vi "1 to 3 Down_movement_v12.vi"(1 "Input pixmap":u8[][](array[numeric]), 2 "start Column":i32) -> (3 "Total point":i32, 4 "moveLog(Row, Col.)":i32[][](array[numeric]), 5 "To:finish Col.":i32, 6 "TapN":dbl)   [LabVIEW 2016]
panel:
  out "RupPoint":dbl[](array[numeric]) format="%_3f"
  out "PointLog":u8[](array[numeric])
  out "min. root p.":u8
  out "3×3 point array":u8[][][](array[numeric])
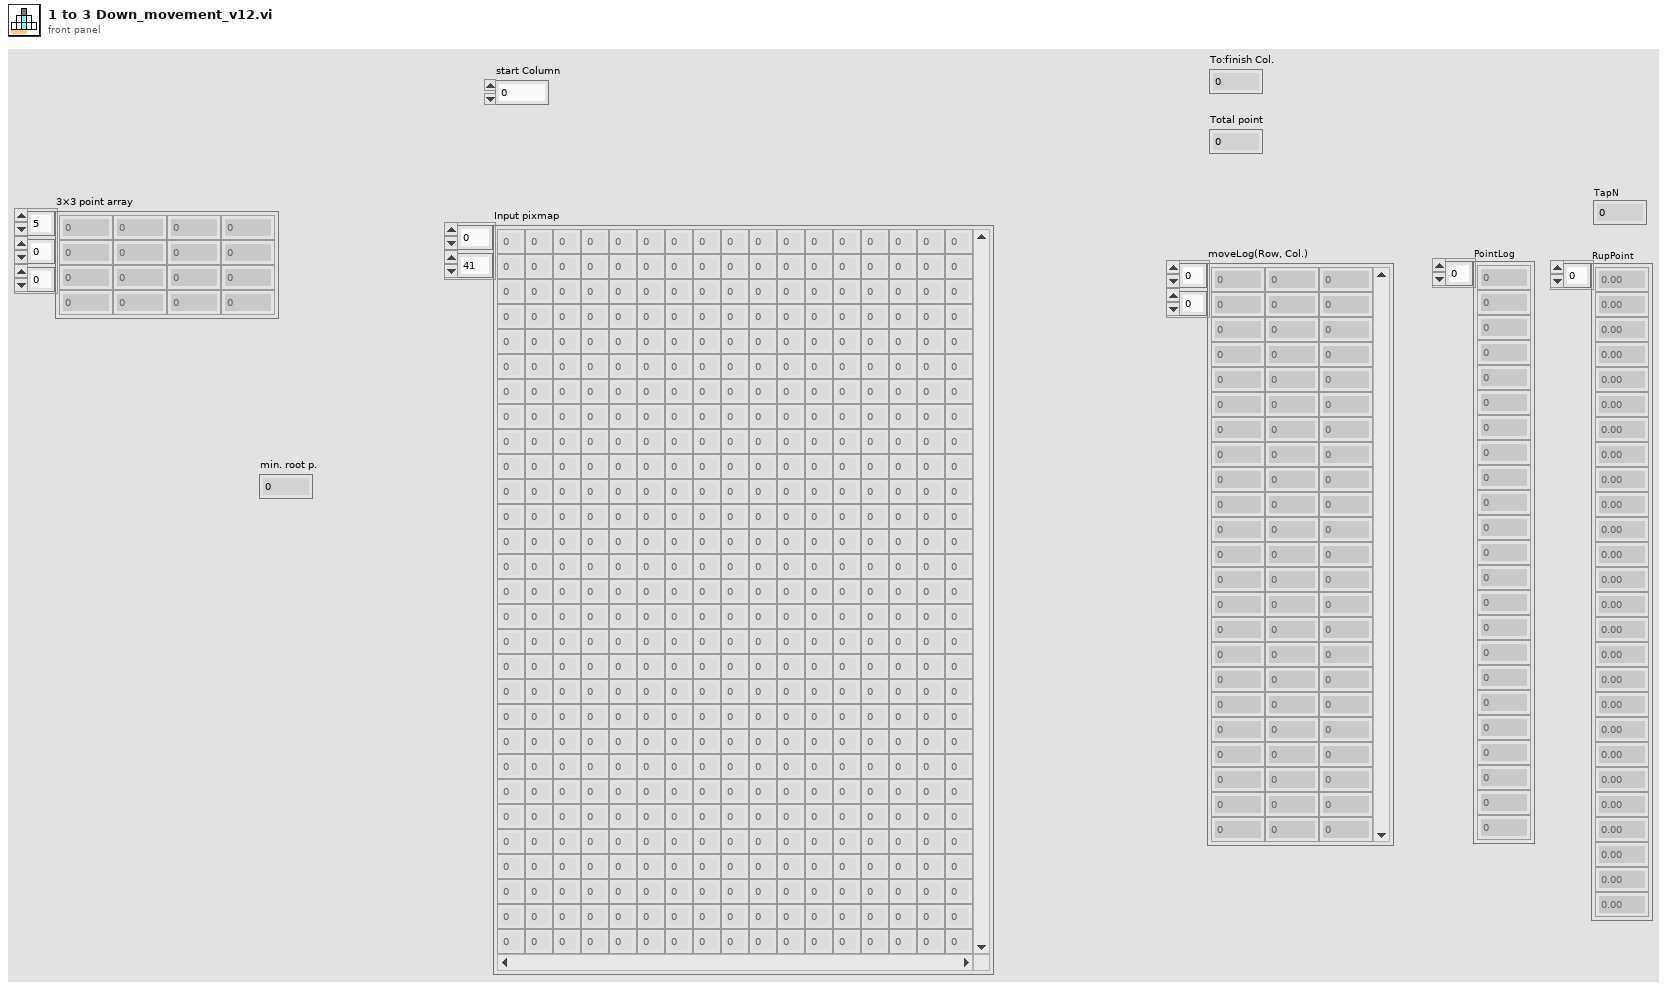
[diagram p1: front panel]
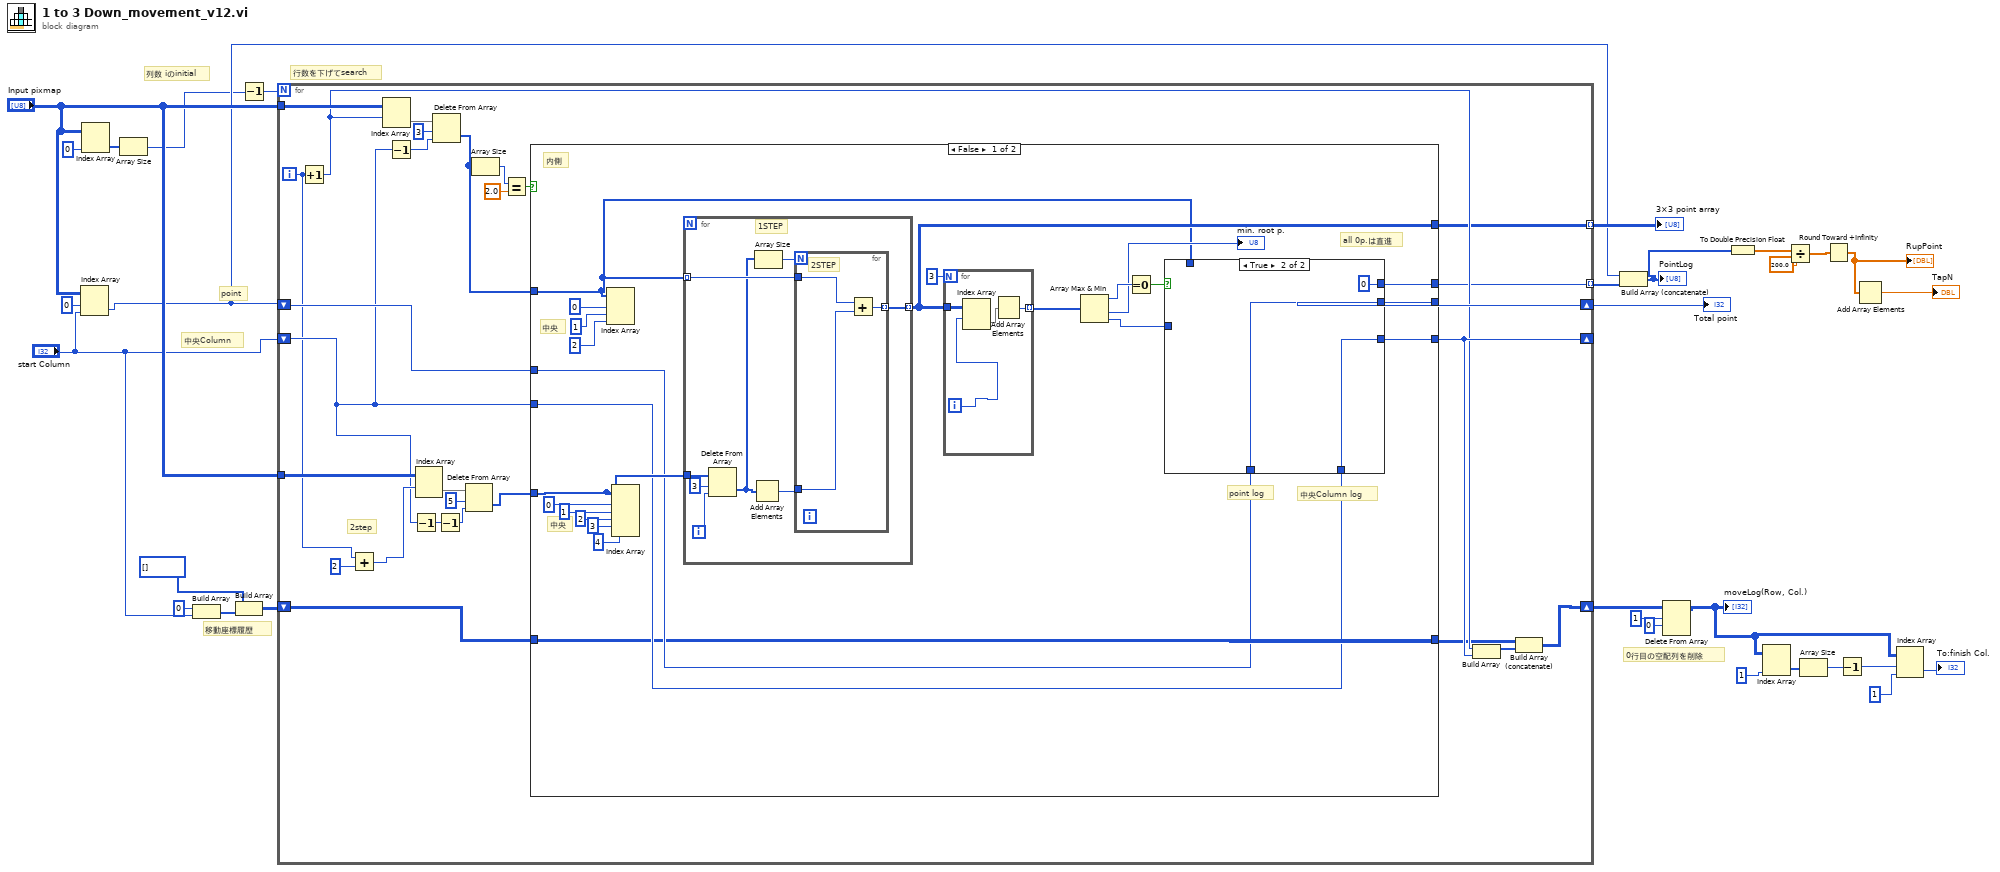
[diagram p0: block diagram]
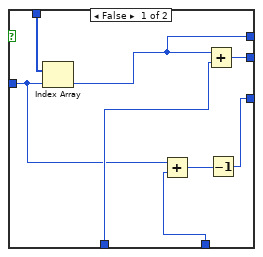
[diagram p2: hidden frame]
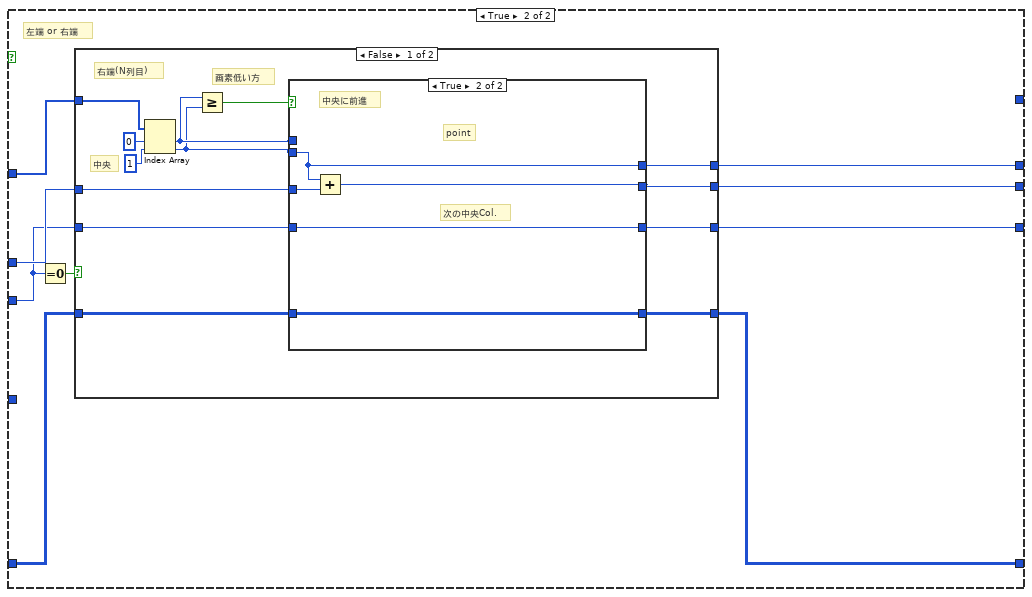
[diagram p3: hidden frame]
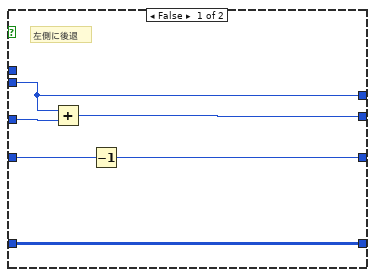
[diagram p4: hidden frame]
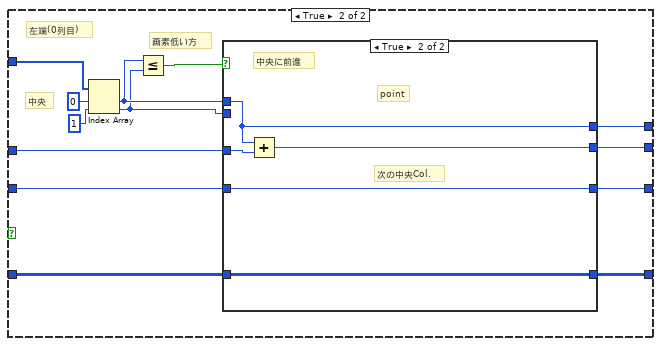
[diagram p5: hidden frame]
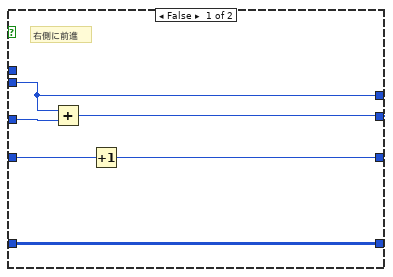
[diagram p6: hidden frame]
diagram:
  # "0行目の空配列を削除"
  # "移動座標履歴"
  # "中央Column"
  # "point"
  # "行数を下げてsearch"
  # "列数 iのinitial"
  n1 = Index Array(array="Input pixmap", index (row)=0 ("無効な指標 （行）"), index (col)="start Column") -> (element=w9:u8)
  n2 = Index Array(array="Input pixmap", index (col)=0 ("無効な指標 （列）")) -> (element=w29:u8[])  [unwired: 1 in]
  n3 = Array Size(array=w29) -> (size(s)=w2:i32)
  n4 = Build Array(0 ("要素"), "start Column") -> (w27:i32[])
  n5 = Build Array(i32[] [] ("要素"), w27) -> (w28:i32[][])
  n6 = Decrement(x=w2) -> (x-1=w1:i32)
  n7 = for {
    N: w1 -> [_]
    tunnel: "Input pixmap" -> [w59]
    shift-right: [w50] -> w31
    shift-left: w9 -> [w51]
    shift-right: [w49] -> _
    shift-left: "start Column" -> [w37]
    shift-right: [w47] -> w25
    shift-left: w28 -> [w48]
    tunnel: "Input pixmap" -> [w39]
    tunnel: [w33] -> w14 mode=indexing
    tunnel: [w32] -> w10 mode=indexing
    i -> [w34]
    # "2step"
    n8 = Increment(x=w34) -> (x+1=w46:i32)
    n9 = Add(x=w34, y=2) -> (x+y=w38:i32)
    n10 = Index Array(array=w59, index (row)=w46) -> (element=w58:u8[])  [unwired: 1 in]
    n11 = Decrement(x=w37) -> (x-1=w56:i32)
    n12 = Decrement(x=w37) -> (x-1=w40:i32)
    n13 = Index Array(array=w39, index (row)=w38) -> (element=w36:u8[])  [unwired: 1 in]
    n14 = Delete From Array(array=w58, length=3 ("長さ"), index=w56) -> (deleted portion=w53:u8[])  [unwired: 1 out]
    n15 = Decrement(x=w40) -> (x-1=w41:i32)
    n16 = Delete From Array(array=w36, length=5 ("長さ"), index=w41) -> (deleted portion=w35:u8[])  [unwired: 1 out]
    n17 = Array Size(array=w53) -> (size(s)=w52:i32)
    n18 = Equal?(x=w52, y=2.0) -> (x = y?=w54:bool)
    n19 = case shown="False" w54 {
      tunnel: w53 -> [w61 w117]
      tunnel: w51 -> [w69 w116]
      tunnel: [w66 w115] -> w50
      tunnel: w37 -> [w68 w112]
      tunnel: [w65 w114] -> w49
      tunnel: [w67 w111] -> w44
      tunnel: w48 -> [w67 w110]
      tunnel: w35 -> [w74 _]
      tunnel: [w64 _] -> w33
      tunnel: [w60 w109] -> w32
      frame False {
        # "中央Column log"
        # "point log"
        # "all 0p.は直進"
        # "中央"
        # "中央"
        # "内側"
        n20 = Index Array(array=w61, index #1=0 ("指標"), index #2=1 ("指標"), index #3=2 ("指標")) -> ()  [unwired: 3 out]
        n21 = Index Array(array=w74, index #1=0 ("指標"), index #2=1 ("指標"), index #3=2 ("指標"), index #4=3 ("指標"), index #5=4 ("指標")) -> ()  [unwired: 5 out]
        n22 = for {
          tunnel: w61 -> [w105] mode=indexing
          tunnel: w74 -> [w103]
          tunnel: [w104] -> w64 mode=indexing
          i -> [w101]
          # "1STEP"
          n23 = Delete From Array(array=w103, length=3 ("長さ"), index=w101) -> (deleted portion=w98:u8[])  [unwired: 1 out]
          n24 = Add Array Elements(numeric array=w98) -> (sum=w99:u8)
          n25 = Array Size(array=w98) -> (size(s)=w100:i32)
          n26 = for {
            N: w100 -> [_]
            tunnel: w105 -> [w108]
            tunnel: [w107] -> w104 mode=indexing
            tunnel: w99 -> [w106]
            # "2STEP"
            n27 = Add(x=w108, y=w106) -> (x+y=w107:u8)
          }
        }
        n28 = for {
          N: 3 -> [_]
          tunnel: w64 -> [w85]
          tunnel: [w86] -> w62 mode=indexing
          i -> [w83]
          n29 = Index Array(array=w85, index (row)=w83) -> (element=w84:u8[])  [unwired: 1 in]
          n30 = Add Array Elements(numeric array=w84) -> (sum=w86:u8)
        }
        n31 = Array Max & Min(array=w62) -> (max value=w72:u8, min value=→"min. root p.":u8, min index (indices)=w73:i32)  [unwired: 1 out]
        n32 = Equal To 0?(x=w72) -> (x = 0?=w71:bool)
        n33 = case shown="True" w71 {
          tunnel: w69 -> [w94 w97]
          tunnel: w73 -> [w88 _]
          tunnel: w68 -> [w92 w96]
          tunnel: [w91 w97] -> w66
          tunnel: [w90 w96] -> w65
          tunnel: w61 -> [w89 _]
          tunnel: [w87 u8 0] -> w60
          frame False {
            n34 = Index Array(array=w89, index=w88) -> (element=w87:u8)
            n35 = Add(x=w88, y=w92) -> (x+y=w93:i32)
            n36 = Add(x=w87, y=w94) -> (x+y=w91:u8)
            n37 = Decrement(x=w93) -> (x-1=w90:i32)
          }
          frame True {
          }
        }
      }
      frame True {
        # "左端 or 右端"
        n38 = Equal To 0?(x=w112) -> (x = 0?=w113:bool)
        n39 = case shown="False" w113 {
          tunnel: w117 -> [w128 w154]
          tunnel: w116 -> [w124 w151]
          tunnel: [w121 w150] -> w115
          tunnel: w112 -> [w123 w149]
          tunnel: [w120 w148] -> w114
          tunnel: [w119 w144] -> w111
          tunnel: w110 -> [w122 w143]
          tunnel: [w118 w142] -> w109
          frame False {
            # "中央"
            # "画素低い方"
            # "右端(N列目)"
            n40 = Index Array(array=w128, index #1=0 ("指標"), index #2=1 ("指標")) -> (element #1=w126:u8, element #2=w125:u8)
            n41 = Greater Or Equal?(x=w126, y=w125) -> (x >= y?=w127:bool)
            n42 = case shown="True" w127 {
              tunnel: w126 -> [_ _]
              tunnel: w124 -> [w132 w141]
              tunnel: [w136 w140] -> w121
              tunnel: w123 -> [w135 w139]
              tunnel: [w134 w139] -> w120
              tunnel: w125 -> [w131 w137]
              tunnel: [w133 w138] -> w119
              tunnel: w122 -> [w133 w138]
              tunnel: [w131 w137] -> w118
              frame False {
                # "左側に後退"
                n43 = Add(x=w131, y=w132) -> (x+y=w136:u8)
                n44 = Decrement(x=w135) -> (x-1=w134:i32)
              }
              frame True {
                # "中央に前進"
                # "次の中央Col."
                # "point"
                n45 = Add(x=w137, y=w141) -> (x+y=w140:u8)
              }
            }
          }
          frame True {
            # "中央"
            # "画素低い方"
            # "左端(0列目)"
            n46 = Index Array(array=w154, index #1=0 ("指標"), index #2=1 ("指標")) -> (element #1=w146:u8, element #2=w145:u8)
            n47 = Less Or Equal?(x=w146, y=w145) -> (x <= y?=w147:bool)
            n48 = case shown="True" w147 {
              tunnel: w146 -> [_ w161]
              tunnel: w151 -> [w160 w165]
              tunnel: [w159 w164] -> w150
              tunnel: w149 -> [w158 w163]
              tunnel: [w157 w163] -> w148
              tunnel: w145 -> [w155 _]
              tunnel: [w156 w162] -> w144
              tunnel: w143 -> [w156 w162]
              tunnel: [w155 w161] -> w142
              frame False {
                # "右側に前進"
                n49 = Add(x=w155, y=w160) -> (x+y=w159:u8)
                n50 = Increment(x=w158) -> (x+1=w157:i32)
              }
              frame True {
                # "中央に前進"
                # "次の中央Col."
                # "point"
                n51 = Add(x=w161, y=w165) -> (x+y=w164:u8)
              }
            }
          }
        }
      }
    }
    n52 = Build Array(w46, w49) -> (w45:i32[])
    n53 = Build Array (concatenate)(w44, w45) -> (w47:i32[][])
  }
  "Total point" <- w31
  "3×3 point array" <- w14
  n54 = Build Array (concatenate)(w9, w10) -> (w5:u8[])
  "PointLog" <- w5
  n55 = Delete From Array(array=w25, length=1 ("長さ"), index (row)=0 ("指標 （行）")) -> (array with subset deleted=w19:i32[][])  [unwired: 1 in, 1 out]
  "moveLog(Row, Col.)" <- w19
  n56 = To Double Precision Float(number=w5) -> (double precision float=w8:dbl[])
  n57 = Index Array(array=w19, index (col)=1 ("指標 （行）")) -> (element=w23:i32[])  [unwired: 1 in]
  n58 = Divide(x=w8, y=200.0) -> (x/y=w6:dbl[])
  n59 = Array Size(array=w23) -> (size(s)=w16:i32)
  n60 = Round Toward +Infinity(x=w6) -> (ceil(x): smallest int >= x=w4:dbl[])
  "RupPoint" <- w4
  n61 = Decrement(x=w16) -> (x-1=w15:i32)
  n62 = Add Array Elements(numeric array=w4) -> (sum=→"TapN":dbl)
  n63 = Index Array(array=w19, index (row)=w15, index (col)=1 ("指標 （行）")) -> (element=→"To:finish Col.":i32)
